vi "ReadData.vi"(8 "Err In":errorcluster, 11 "TCP In":refnum<class "TCP.lvclass">) -> (0 "Err Out":errorcluster, 1 "read buffer":string, 3 "TCP Out":refnum<class "TCP.lvclass">)   [LabVIEW 2019, in "TCP.lvclass"]
uses:
  TCP.lvclass
  TCP.lvclass/TCP.ctl
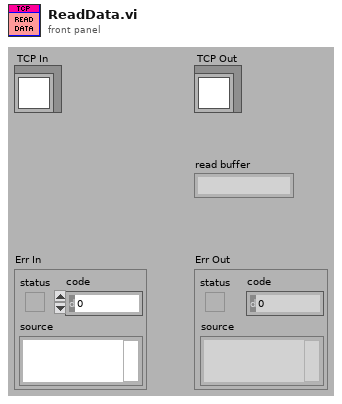
[diagram p1: front panel]
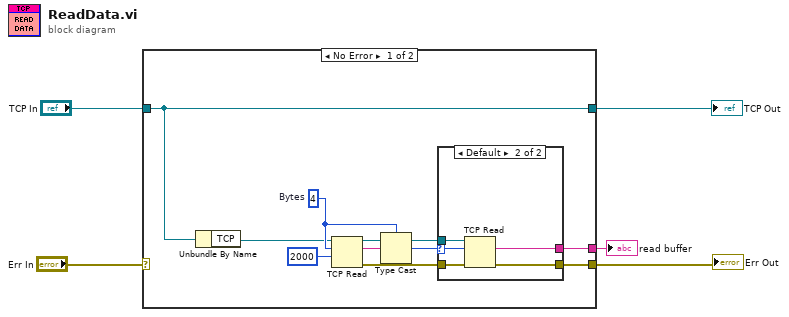
[diagram p0: block diagram]
diagram:
  n1 = case shown="No Error" "Err In" {
    selector: "Err In" -> [_ w23]
    tunnel: [w7 w23] -> w4
    tunnel: [w15 w22] -> w2
    tunnel: "TCP In" -> [w15 w22]
    tunnel: [w6 _] -> w1
    frame No Error {
      w11 = 4  # Bytes
      n2 = Unbundle By Name(w15) -> ("TCP"=w8:refnum<k5>)
      n3 = TCP Read(connection ID=w8, bytes to read=w11, 9:2000 ("timeout ms (25000)")) -> (connection ID out=w13:refnum<k5>, data out=w14:string, error out=w12:errorcluster)  [unwired: 2 in]
      n4 = Type Cast(type=w11, x=w14) -> (*(type *) &x=w10:i32)
      n5 = case shown="Default" w10 {
        selector: w10 -> [_ w18]
        tunnel: w13 -> [_ w21]
        tunnel: w12 -> [w16 w20]
        tunnel: [w16 w19] -> w7
        tunnel: [_ w17] -> w6
        frame ..0 {
        }
        frame Default {
          n6 = TCP Read(connection ID=w21, bytes to read=w18, error in (no error)=w20) -> (data out=w17:string, error out=w19:errorcluster)  [unwired: 2 in, 1 out]
        }
      }
    }
    frame Error {
    }
  }
  "Err Out" <- w4
  "TCP Out" <- w2
  "read buffer" <- w1
